vi "Get State.vi"(8 "error in (no error)":errorcluster, 11 "Micron sm Digitizer in":refnum<class "Micron sm Digitizer.lvclass">) -> (0 "error out":errorcluster, 1 "Data ready":bool, 2 "Armed":bool, 3 "Micron sm Digitizer out":refnum<class "Micron sm Digitizer.lvclass">, 4 "Availiable Samples":u32, 5 "Finished":bool)   [LabVIEW 2024, in "Micron sm Digitizer.lvclass"]
uses:
  Micron sm Digitizer.lvclass
  Micron sm Digitizer.lvclass/Micron sm Digitizer.ctl
  Strain/Micron Optics sm130/Micron Optics sm130.lvlib
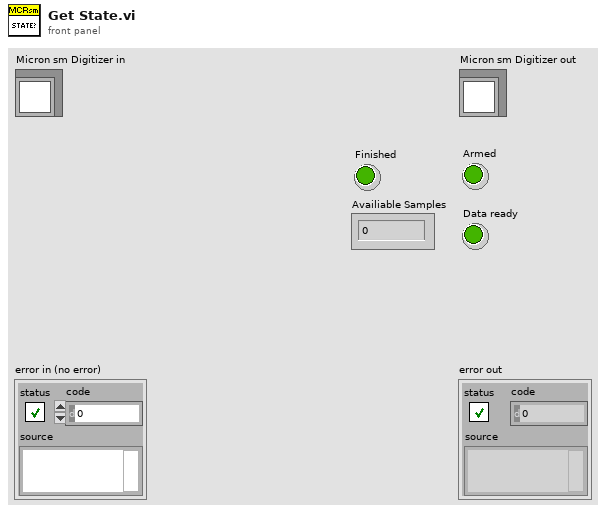
[diagram p1: front panel]
types:
  T1 = typedef "Micron optics didgitizer configuration.ctl" = cluster{"Post-trigger delay":dbl, "Post-trigger duration":dbl, "Rate":dbl, "Ranges":dbl[], "Re-name channels":string[], "Active channels":string, "External\nclock":bool, "Reference channel":i32, "Detection Setting IDs":u8[], "Stream and average":bool, "Address":string, "Number of sensors":i32}
  T2 = cluster{"Full Spectrum Radix":u8, "Firmware Version":u8, "Primary Fan":bool, "Secondary Fan":bool, "Switch Position":u8, "MUX":u8, "Trigger Mode":u8, "Operating Mode":u8, "Data Serial Number":u32, "Time Stamp":dbl, "Buffer (%)":u8, "MUX Level":u8}
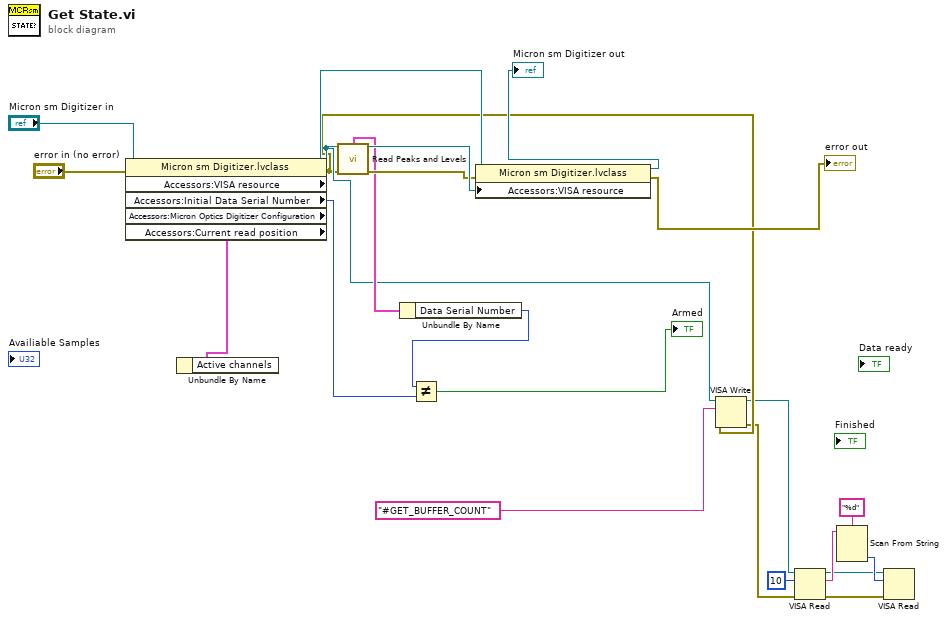
[diagram p0: block diagram]
diagram:
  n1 = property class="Micron sm Digitizer.lvclass" props=["Accessors:VISA resource", "Accessors:Initial Data Serial Number", "Accessors:Micron Optics Digitizer Configuration", "Accessors:Current read position"](reference="Micron sm Digitizer in", error in="error in (no error)") -> (reference out=w19:refnum<class "Micron sm Digitizer.lvclass">, error out=w9:errorcluster, "Accessors:VISA resource"=w10:refnum<visa-resource-name>, "Accessors:Initial Data Serial Number"=w12:u32, "Accessors:Micron Optics Digitizer Configuration"=w13:T1)  [unwired: 1 out]
  n2 = Unbundle By Name(w13) -> ()  [unwired: 1 out]
  n3 = call "Read Peaks and Levels.vi"("VISA resource name"=w10, "error in (no error)"=w9) -> ("Status"=w16:T2, "VISA resource name out"=w21:refnum<visa-resource-name>, "error out"=w20:errorcluster)  [unwired: 5 in, 6 out]
  n4 = Unbundle By Name(w16) -> ("Data Serial Number"=w15:u32)
  n5 = Not Equal?(x=w15, y=w12) -> (x != y?=→"Armed":bool)
  n6 = property class="Micron sm Digitizer.lvclass"(reference=w19, error in=w20, "Accessors:VISA resource"=w21) -> (reference out=→"Micron sm Digitizer out":refnum<class "Micron sm Digitizer.lvclass">, error out=→"error out":errorcluster)
  n7 = VISA Write(VISA resource name=w10, write buffer="#GET_BUFFER_COUNT" ("string"), error in (no error)=w9) -> (VISA resource name out=w2:refnum<visa-resource-name>, error out=w1:errorcluster)  [unwired: 1 out]
  n8 = VISA Read(VISA resource name=w2, byte count=u32 10, error in (no error)=w1) -> (VISA resource name out=w3:refnum<visa-resource-name>, read buffer=w6:string, error out=w4:errorcluster)  [unwired: 1 out]
  n9 = Scan From String(format string="%d", input string=w6) -> (output 1=w7:i32)  [unwired: 3 in, 3 out]
  n10 = VISA Read(VISA resource name=w3, byte count=w7, error in (no error)=w4) -> ()  [unwired: 4 out]
